vi "Close Scalar Refs.vi"(8 "error in (no error)":errorcluster, 11 "Cluster":T1 {"Data Type" format="%.0x"}) -> (0 "error out":errorcluster)   [LabVIEW 2016, in "FPGA Addon Engine.lvlib"]
uses:
  FPGA Addon Engine.lvlib
  Types/Register Settings.ctl
  FPGA-Resource-Manager-APIs/Source/Shared/Types/Data Type.ctl
  FPGA-Resource-Manager-APIs/Source/Shared/Types/Scalar Type.ctl
  <vilib>/FPGAPlugInAG/Dynamic/niLvFpga_Close_Dynamic.vi
  <vilib>/rvi/interface/nirviCloseFPGA/nirviCloseFPGA.xnode
  FPGA-Resource-Manager-APIs/Source/Shared/FPGA RM Shared API.lvlib
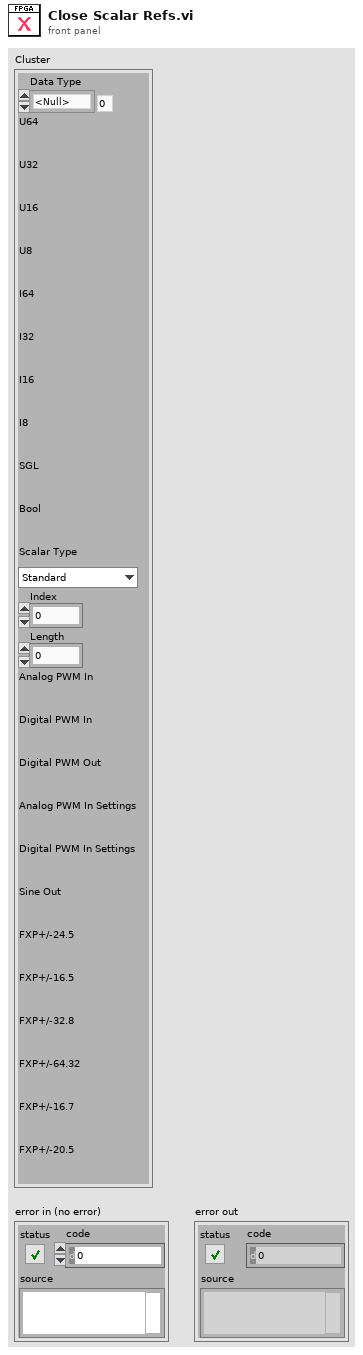
[diagram p1: front panel]
types:
  T1 = typedef "FPGA Addon Engine.lvlib/Register Settings.ctl" = cluster{"Data Type":T2, "U64":refnum<k20>, "U32":refnum<k20>, "U16":refnum<k20>, "U8":refnum<k20>, "I64":refnum<k20>, "I32":refnum<k20>, "I16":refnum<k20>, "I8":refnum<k20>, "SGL":refnum<k20>, "Bool":refnum<k20>, "Scalar Type":T3, "Index":i32, "Length":i32, "Analog PWM In":refnum<k20>, "Digital PWM In":refnum<k20>, "Digital PWM Out":refnum<k20>, "Analog PWM In Settings":refnum<k20>, "Digital PWM In Settings":refnum<k20>, "Sine Out":refnum<k20>, "FXP+/-24.5":refnum<k20>, "FXP+/-16.5":refnum<k20>, "FXP+/-32.8":refnum<k20>, "FXP+/-64.32":refnum<k20>, "FXP+/-16.7":refnum<k20>, "FXP+/-20.5":refnum<k20>}
  T2 = typedef "FPGA RM Shared API.lvlib/Data Type.ctl" = enum8{"<Null>", "I8", "I16", "I32", "I64", "U8", "U16", "U32", "U64", "SGL", "Boolean", "Analog PWM In Settings", "Analog PWM In", "Digital PWM In Settings", "Digital PWM In", "Digital PWM Out", "Sine Out", "FXP+/-24.5", "FXP+/-16.5", "FXP+/-32.8", "FXP+/-64.32", "FXP+/-16.7", "FXP+/-20.5"}
  T3 = typedef "FPGA RM Shared API.lvlib/Scalar Type.ctl" = enum16{"Standard", "Bitpacked"}
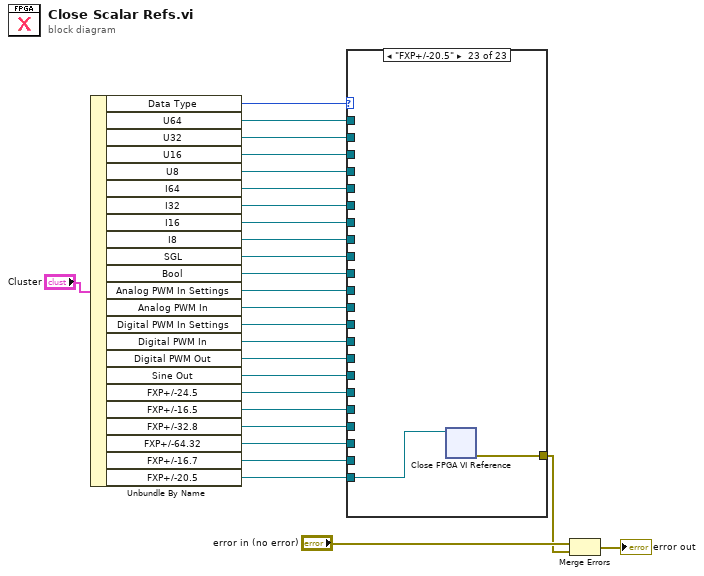
[diagram p0: block diagram]
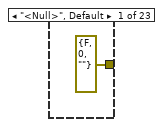
[diagram p2: hidden frame]
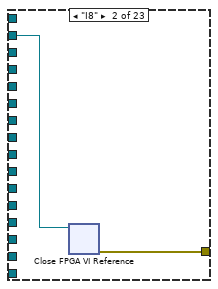
[diagram p3: hidden frame]
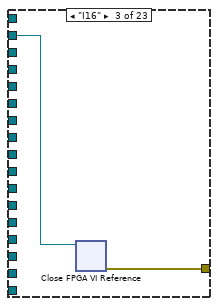
[diagram p4: hidden frame]
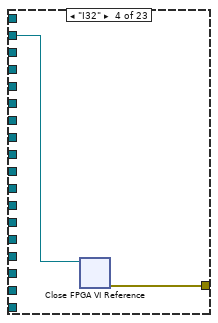
[diagram p5: hidden frame]
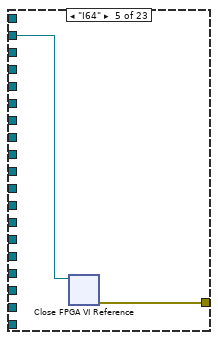
[diagram p6: hidden frame]
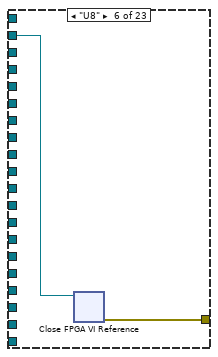
[diagram p7: hidden frame]
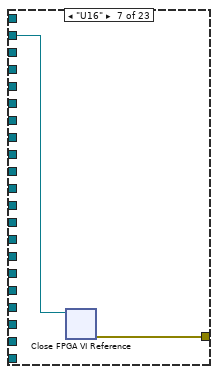
[diagram p8: hidden frame]
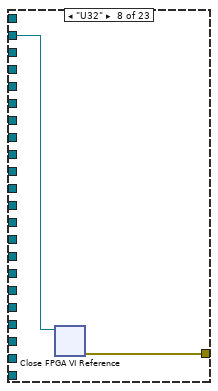
[diagram p9: hidden frame]
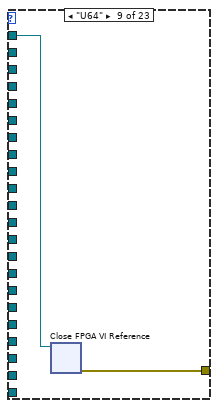
[diagram p10: hidden frame]
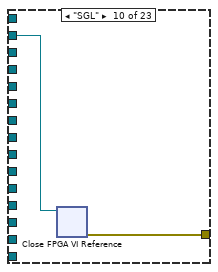
[diagram p11: hidden frame]
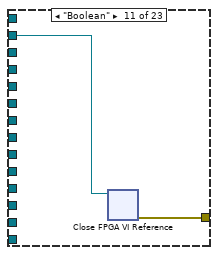
[diagram p12: hidden frame]
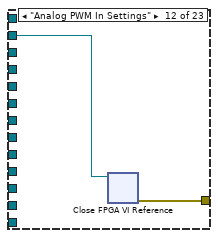
[diagram p13: hidden frame]
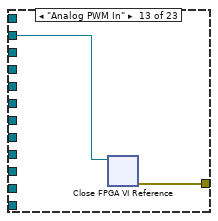
[diagram p14: hidden frame]
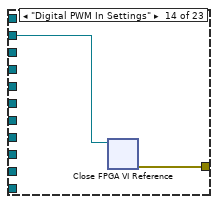
[diagram p15: hidden frame]
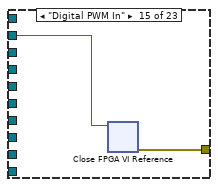
[diagram p16: hidden frame]
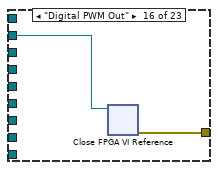
[diagram p17: hidden frame]
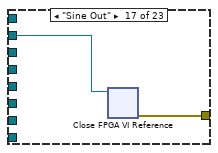
[diagram p18: hidden frame]
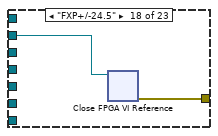
[diagram p19: hidden frame]
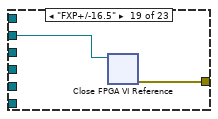
[diagram p20: hidden frame]
diagram:
  n1 = Unbundle By Name("Cluster") -> ("Data Type"=w27:T2, "U64"=w16:refnum<k20>, "U32"=w17:refnum<k20>, "U16"=w18:refnum<k20>, "U8"=w19:refnum<k20>, "I64"=w20:refnum<k20>, "I32"=w21:refnum<k20>, "I16"=w22:refnum<k20>, "I8"=w26:refnum<k20>, "SGL"=w24:refnum<k20>, "Bool"=w23:refnum<k20>, "Analog PWM In Settings"=w2:refnum<k20>, "Analog PWM In"=w3:refnum<k20>, "Digital PWM In Settings"=w4:refnum<k20>, "Digital PWM In"=w5:refnum<k20>, "Digital PWM Out"=w6:refnum<k20>, "Sine Out"=w7:refnum<k20>, "FXP+/-24.5"=w8:refnum<k20>, "FXP+/-16.5"=w9:refnum<k20>, "FXP+/-32.8"=w10:refnum<k20>, "FXP+/-64.32"=w11:refnum<k20>, "FXP+/-16.7"=w12:refnum<k20>, "FXP+/-20.5"=w1:refnum<k20>)
  n2 = case shown="\"FXP+/-20.5\"" w27 {
    tunnel: w26 -> [_ w29 _ _ _ _ _ _ _ _ _ _ _ _ _ _ _ _ _ _ _ _ _]
    tunnel: [errorcluster {"status"=FALSE, "code"=0, "source"=""} ("error out") w30 w32 w34 w36 w38 w40 w42 w44 w45 w48 w50 w52 w54 w56 w58 w60 w62 w64 w66 w68 w70 w72] -> w14
    tunnel: w24 -> [_ _ _ _ _ _ _ _ _ w46 _ _ _ _ _ _ _ _ _ _ _ _ _]
    tunnel: w23 -> [_ _ _ _ _ _ _ _ _ _ w47 _ _ _ _ _ _ _ _ _ _ _ _]
    tunnel: w22 -> [_ _ w31 _ _ _ _ _ _ _ _ _ _ _ _ _ _ _ _ _ _ _ _]
    tunnel: w21 -> [_ _ _ w33 _ _ _ _ _ _ _ _ _ _ _ _ _ _ _ _ _ _ _]
    tunnel: w20 -> [_ _ _ _ w35 _ _ _ _ _ _ _ _ _ _ _ _ _ _ _ _ _ _]
    tunnel: w19 -> [_ _ _ _ _ w37 _ _ _ _ _ _ _ _ _ _ _ _ _ _ _ _ _]
    tunnel: w18 -> [_ _ _ _ _ _ w39 _ _ _ _ _ _ _ _ _ _ _ _ _ _ _ _]
    tunnel: w17 -> [_ _ _ _ _ _ _ w41 _ _ _ _ _ _ _ _ _ _ _ _ _ _ _]
    tunnel: w16 -> [_ _ _ _ _ _ _ _ w43 _ _ _ _ _ _ _ _ _ _ _ _ _ _]
    tunnel: w12 -> [_ _ _ _ _ _ _ _ _ _ _ _ _ _ _ _ _ _ _ _ _ w69 _]
    tunnel: w11 -> [_ _ _ _ _ _ _ _ _ _ _ _ _ _ _ _ _ _ _ _ w67 _ _]
    tunnel: w10 -> [_ _ _ _ _ _ _ _ _ _ _ _ _ _ _ _ _ _ _ w65 _ _ _]
    tunnel: w9 -> [_ _ _ _ _ _ _ _ _ _ _ _ _ _ _ _ _ _ w63 _ _ _ _]
    tunnel: w8 -> [_ _ _ _ _ _ _ _ _ _ _ _ _ _ _ _ _ w61 _ _ _ _ _]
    tunnel: w7 -> [_ _ _ _ _ _ _ _ _ _ _ _ _ _ _ _ w59 _ _ _ _ _ _]
    tunnel: w6 -> [_ _ _ _ _ _ _ _ _ _ _ _ _ _ _ w57 _ _ _ _ _ _ _]
    tunnel: w5 -> [_ _ _ _ _ _ _ _ _ _ _ _ _ _ w55 _ _ _ _ _ _ _ _]
    tunnel: w4 -> [_ _ _ _ _ _ _ _ _ _ _ _ _ w53 _ _ _ _ _ _ _ _ _]
    tunnel: w3 -> [_ _ _ _ _ _ _ _ _ _ _ _ w51 _ _ _ _ _ _ _ _ _ _]
    tunnel: w2 -> [_ _ _ _ _ _ _ _ _ _ _ w49 _ _ _ _ _ _ _ _ _ _ _]
    tunnel: w1 -> [_ _ _ _ _ _ _ _ _ _ _ _ _ _ _ _ _ _ _ _ _ _ w71]
    frame "<Null>", Default {
    }
    frame "I8" {
      n3 = xnode "Close FPGA VI Reference"("FPGA VI Reference In"=w29) -> ("error out"=w30:errorcluster)  [unwired: 1 in]
    }
    frame "I16" {
      n4 = xnode "Close FPGA VI Reference"("FPGA VI Reference In"=w31) -> ("error out"=w32:errorcluster)  [unwired: 1 in]
    }
    frame "I32" {
      n5 = xnode "Close FPGA VI Reference"("FPGA VI Reference In"=w33) -> ("error out"=w34:errorcluster)  [unwired: 1 in]
    }
    frame "I64" {
      n6 = xnode "Close FPGA VI Reference"("FPGA VI Reference In"=w35) -> ("error out"=w36:errorcluster)  [unwired: 1 in]
    }
    frame "U8" {
      n7 = xnode "Close FPGA VI Reference"("FPGA VI Reference In"=w37) -> ("error out"=w38:errorcluster)  [unwired: 1 in]
    }
    frame "U16" {
      n8 = xnode "Close FPGA VI Reference"("FPGA VI Reference In"=w39) -> ("error out"=w40:errorcluster)  [unwired: 1 in]
    }
    frame "U32" {
      n9 = xnode "Close FPGA VI Reference"("FPGA VI Reference In"=w41) -> ("error out"=w42:errorcluster)  [unwired: 1 in]
    }
    frame "U64" {
      n10 = xnode "Close FPGA VI Reference"("FPGA VI Reference In"=w43) -> ("error out"=w44:errorcluster)  [unwired: 1 in]
    }
    frame "SGL" {
      n11 = xnode "Close FPGA VI Reference"("FPGA VI Reference In"=w46) -> ("error out"=w45:errorcluster)  [unwired: 1 in]
    }
    frame "Boolean" {
      n12 = xnode "Close FPGA VI Reference"("FPGA VI Reference In"=w47) -> ("error out"=w48:errorcluster)  [unwired: 1 in]
    }
    frame "Analog PWM In Settings" {
      n13 = xnode "Close FPGA VI Reference"("FPGA VI Reference In"=w49) -> ("error out"=w50:errorcluster)  [unwired: 1 in]
    }
    frame "Analog PWM In" {
      n14 = xnode "Close FPGA VI Reference"("FPGA VI Reference In"=w51) -> ("error out"=w52:errorcluster)  [unwired: 1 in]
    }
    frame "Digital PWM In Settings" {
      n15 = xnode "Close FPGA VI Reference"("FPGA VI Reference In"=w53) -> ("error out"=w54:errorcluster)  [unwired: 1 in]
    }
    frame "Digital PWM In" {
      n16 = xnode "Close FPGA VI Reference"("FPGA VI Reference In"=w55) -> ("error out"=w56:errorcluster)  [unwired: 1 in]
    }
    frame "Digital PWM Out" {
      n17 = xnode "Close FPGA VI Reference"("FPGA VI Reference In"=w57) -> ("error out"=w58:errorcluster)  [unwired: 1 in]
    }
    frame "Sine Out" {
      n18 = xnode "Close FPGA VI Reference"("FPGA VI Reference In"=w59) -> ("error out"=w60:errorcluster)  [unwired: 1 in]
    }
    frame "FXP+/-24.5" {
      n19 = xnode "Close FPGA VI Reference"("FPGA VI Reference In"=w61) -> ("error out"=w62:errorcluster)  [unwired: 1 in]
    }
    frame "FXP+/-16.5" {
      n20 = xnode "Close FPGA VI Reference"("FPGA VI Reference In"=w63) -> ("error out"=w64:errorcluster)  [unwired: 1 in]
    }
    frame "FXP+/-32.8" {
      n21 = xnode "Close FPGA VI Reference"("FPGA VI Reference In"=w65) -> ("error out"=w66:errorcluster)  [unwired: 1 in]
    }
    frame "FXP+/-64.32" {
      n22 = xnode "Close FPGA VI Reference"("FPGA VI Reference In"=w67) -> ("error out"=w68:errorcluster)  [unwired: 1 in]
    }
    frame "FXP+/-16.7" {
      n23 = xnode "Close FPGA VI Reference"("FPGA VI Reference In"=w69) -> ("error out"=w70:errorcluster)  [unwired: 1 in]
    }
    frame "FXP+/-20.5" {
      n24 = xnode "Close FPGA VI Reference"("FPGA VI Reference In"=w71) -> ("error out"=w72:errorcluster)  [unwired: 1 in]
    }
  }
  n25 = Merge Errors("error in (no error)", w14) -> (→"error out":errorcluster)
